vi "Initialize.vi"(8 "error in (no error)":errorcluster, 11 "MeasurementServiceV1 in":refnum<class "MeasurementServiceV1.lvclass">) -> (0 "error out":errorcluster, 3 "MeasurementServiceV1 out":refnum<class "MeasurementServiceV1.lvclass">)   [LabVIEW 2020, in "MeasurementLink Measurement Server.lvlib" / "MeasurementServiceV1.lvclass"]
uses:
  MeasurementServiceV1.lvclass
  MeasurementLink Measurement Server Internal/RPC Service/MeasurementService/MeasurementService.lvclass
  MeasurementServiceV1.lvclass/MeasurementServiceV1.ctl
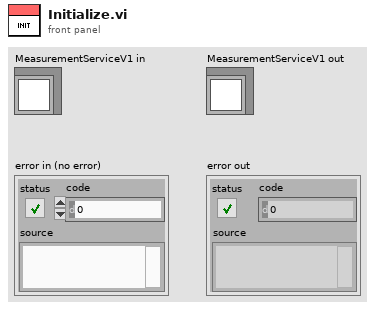
[diagram p1: front panel]
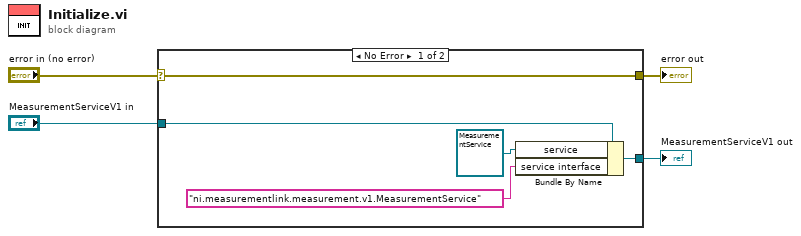
[diagram p0: block diagram]
diagram:
  n1 = case shown="No Error" "error in (no error)" {
    selector: "error in (no error)" -> [w9 w10]
    tunnel: [w9 w10] -> w3
    tunnel: "MeasurementServiceV1 in" -> [w8 w11]
    tunnel: [w5 w11] -> w1
    frame No Error {
      n2 = Bundle By Name(cluster=w8, "service"=refnum<class "MeasurementService.lvclass"> refnum, "service interface"="ni.measurementlink.measurement.v1.MeasurementService") -> (w5:refnum<class "MeasurementServiceV1.lvclass">)
    }
    frame Error {
    }
  }
  "MeasurementServiceV1 out" <- w1
  "error out" <- w3
